vi "Main.vi"(11 "Module Admin":refnum<class "Delacor_lib_QMH_Cloneable Module Admin.lvclass">) -> ()   [LabVIEW 2020, in "TCP Client.lvlib"]
doc: "This template is based off of the Queued Message Handler design pattern and the Queued Message Handler project template that ships with LabVIEW.\n\nThe main difference is that the queue is private to this module and communication between modules is performed via Broadcast and Request events.\n\nRequest events are wrapped in public API methods and are handled in the Event Handling Loop (EHL) of this VI. Any module can register for Broadcast events sent by this module. The EHL generates messages based on user interface actions.\n\nThe Message Handling Loop (MHL) processes messages generated by the EHL, or by other messages. The messages are string values, so new messages can be added easily to the Message Cases case structure in the MHL. Each message cluster can also provide an optional value for Message Data, which is a variant that can be converted to whatever message-specific data is required.\n_____\nBased on Delacor QMH Project Template 6.0.0.89."
uses:
  TCP Client.lvlib
  <vilib>/Delacor/Delacor QMH/Libraries/Cloneable Module Admin_class/Delacor_lib_QMH_Cloneable Module Admin.lvclass
  C:/Program Files (x86)/National Instruments/LabVIEW 2020/vi.lib/Delacor/Delacor QMH/Libraries/Module Admin_class/Delacor_lib_QMH_Module Admin.lvclass
  Module Data--cluster.ctl
  <vilib>/Delacor/Delacor QMH/Libraries/Cloneable Module Admin_class/Delacor_lib_QMH_Cloneable Module Admin.lvclass/Delacor_lib_QMH_Cloneable Module Admin.ctl
  Stop Argument--cluster.ctl
  <vilib>/Delacor/Delacor QMH/Libraries/Message Queue_class/Delacor_lib_QMH_Message Queue.lvclass/Delacor_lib_QMH_Message Queue.ctl
  <vilib>/Delacor/Delacor QMH/Libraries/Module Admin_class/Delacor_lib_QMH_Module Admin.lvclass/Delacor_lib_QMH_Module Admin.ctl
  <vilib>/Utility/miscctls.llb/LVPointTypeDef.ctl
  <vilib>/Delacor/Delacor QMH/Libraries/Cloneable Module Admin_class/Delacor_lib_QMH_Get Module ID.vi
  <vilib>/Delacor/Delacor QMH/Libraries/Message Queue_class/Delacor_lib_QMH_Enqueue Message (Single).vi
  <vilib>/Delacor/Delacor QMH/Libraries/Module Admin_class/Delacor_lib_QMH_Get External Launch.vi
  <vilib>/Utility/error.llb/Error Cluster From Error Code.vi
  <vilib>/ErrorRing/Error Ring.xnode
  <vilib>/Delacor/Delacor QMH/Libraries/Message Queue_class/Delacor_lib_QMH_Message Queue.lvclass
  Test TCP Server API/TCP Server.lvlib
panel:
  out "Module ID":i32=-1
  out "# of Connections":i32
  out "Recieve":T1 {"Gauge" scale=0.0..10.0; "Slide" scale=0.0..10.0}
  out "error out":errorcluster
  out "Status":string
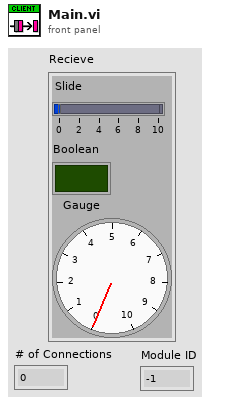
[diagram p1: front panel]
types:
  T1 = cluster{"Slide":dbl, "Boolean":bool, "Gauge":dbl}
  T2 = typedef "TCP Client.lvlib/Request Events--cluster.ctl" = cluster{"Stop Module":refnum<user-event>, "Show Panel":refnum<user-event>, "Hide Panel":refnum<user-event>, "Show Diagram":refnum<user-event>, "Get Module Execution Status":refnum<user-event>, "Connect to TCP Server":refnum<user-event>}
  T3 = typedef "TCP Server.lvlib/Broadcast Events--cluster.ctl" = cluster{"Module Did Init":refnum<user-event>, "Status Updated":refnum<user-event>, "Error Reported":refnum<user-event>, "Module Did Stop":refnum<user-event>, "Update Module Execution Status":refnum<user-event>, "module number":refnum<user-event>}
  T4 = typedef "TCP Client.lvlib/Module Data--cluster.ctl" = cluster{"Status":string}
  T5 = enum32{"invalid lock state", "Not Locked", "Locked (No Password)", "Password-protected"}
  T6 = typedef "TCP Client.lvlib/Stop Argument--cluster.ctl" = cluster{"Module ID":i32, "Origin":string, "Exit via Stop Module Req?":bool, "Wait for Module to stop?":bool}
  T7 = typedef "LVPointTypeDef.ctl" = cluster{"Horizontal":i16, "Vertical":i16}
  T8 = enum32{"Invalid", "Standard", "Closed", "Hidden", "Minimized", "Maximized"}
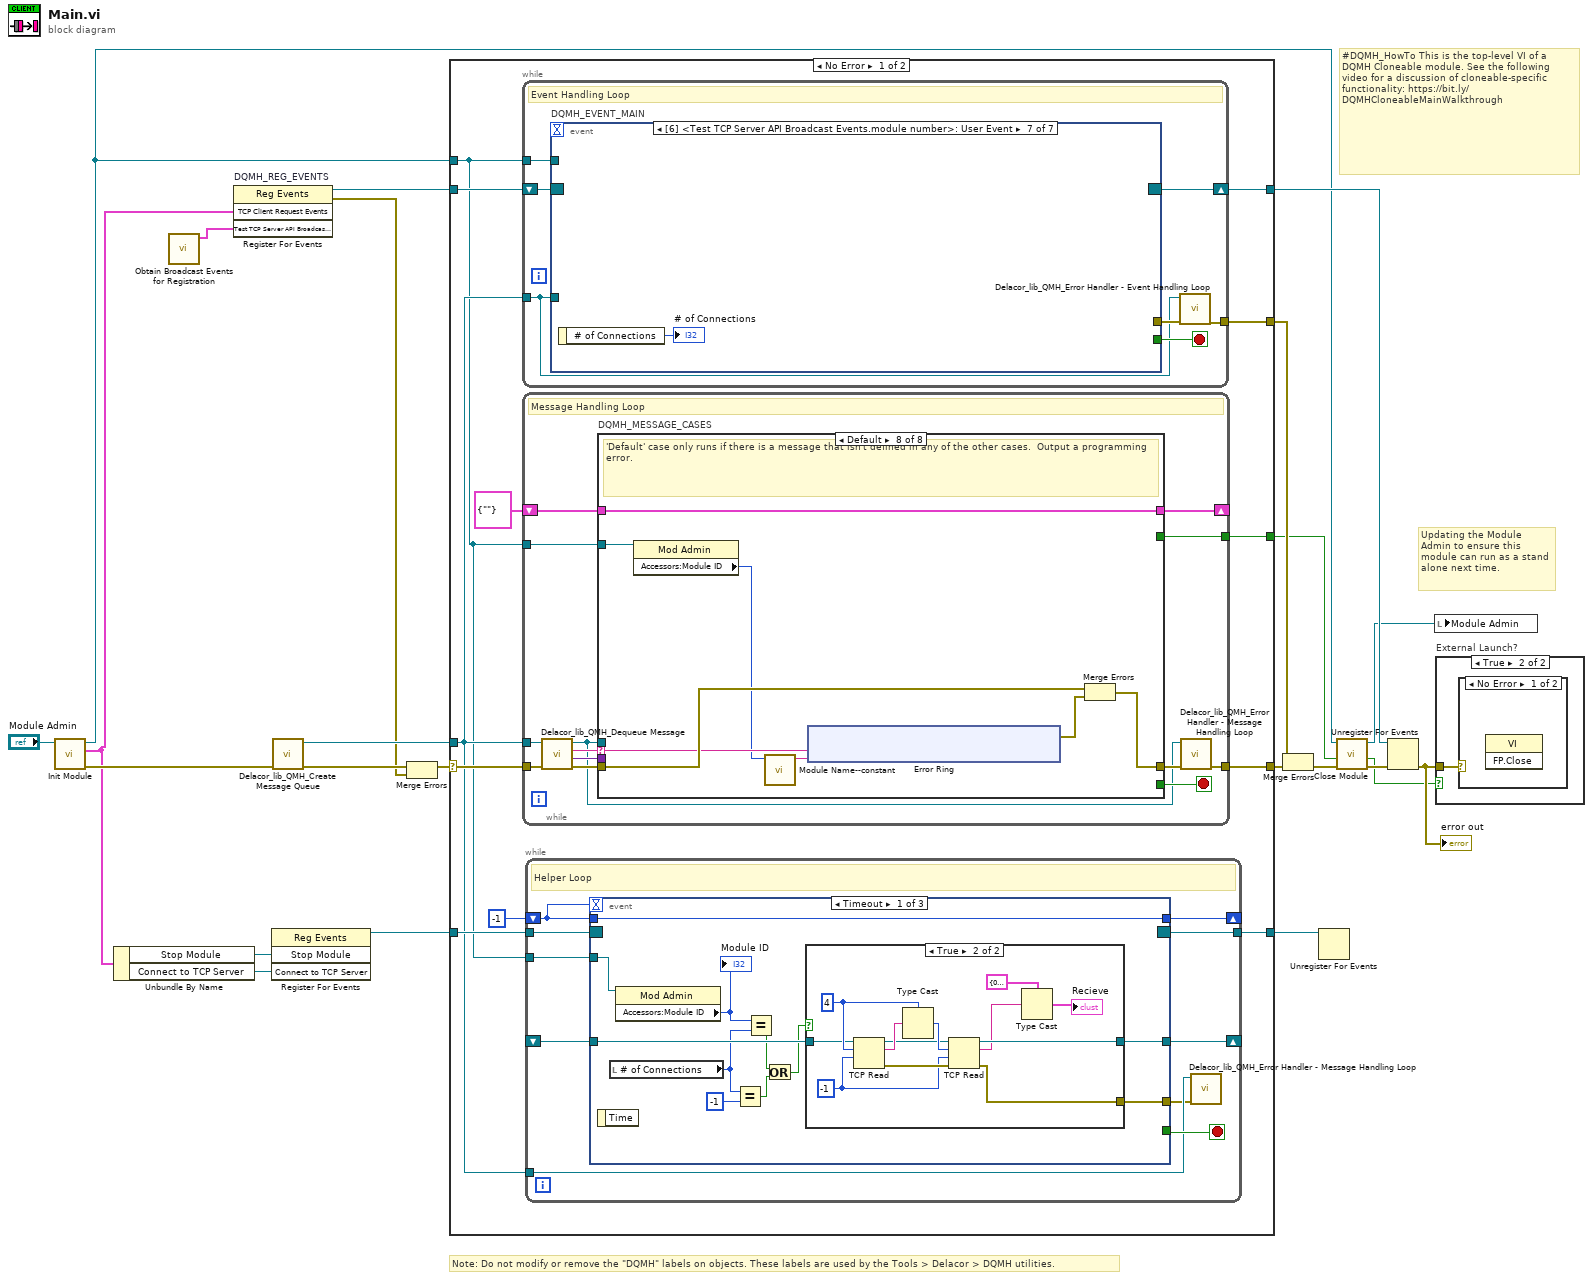
[diagram p0: block diagram]
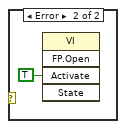
[diagram p3: hidden frame]
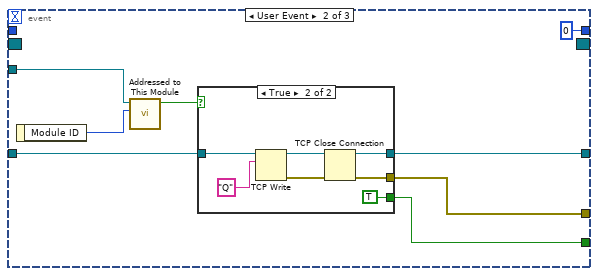
[diagram p5: hidden frame]
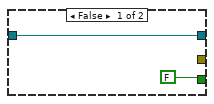
[diagram p6: hidden frame]
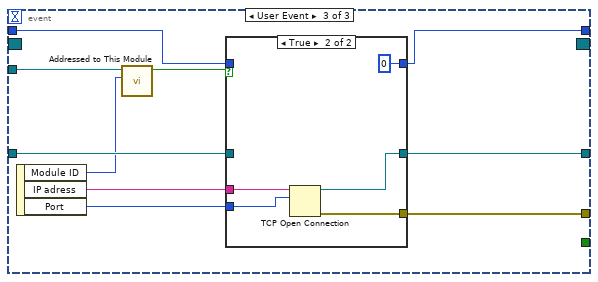
[diagram p7: hidden frame]
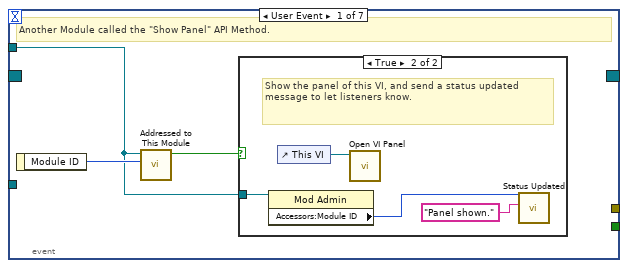
[diagram p9: hidden frame]
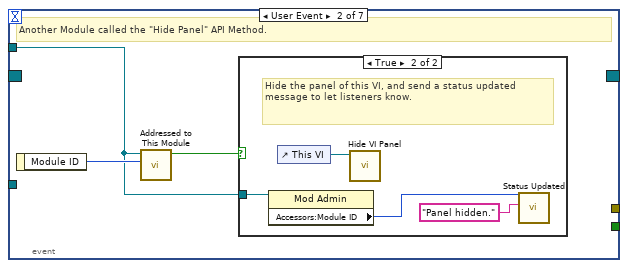
[diagram p11: hidden frame]
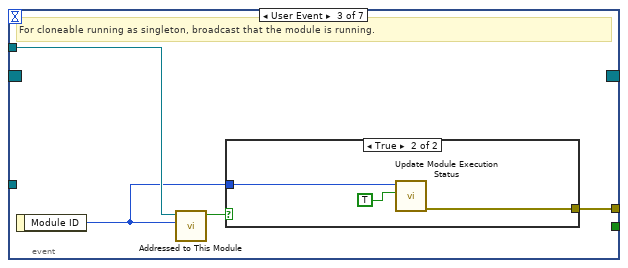
[diagram p13: hidden frame]
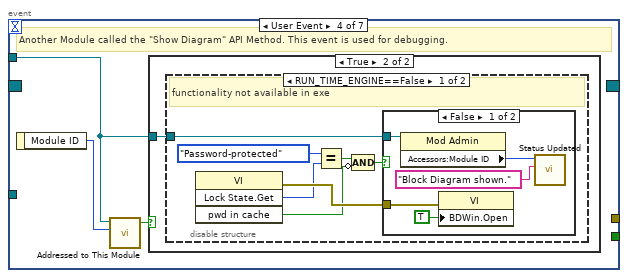
[diagram p15: hidden frame]
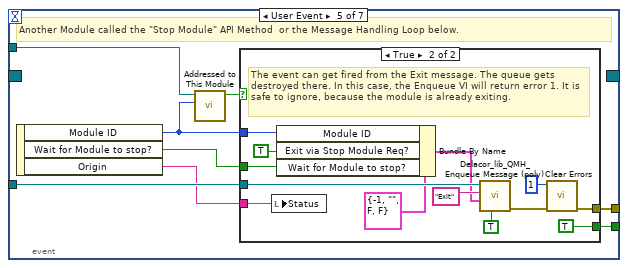
[diagram p19: hidden frame]
diagram:
  # "#DQMH_HowTo This is the top-level VI of a DQMH Cloneable module. See the following video for a discussion of cloneable-specific functionality: https://bit.ly/DQMHCloneableMainWalkthrough"
  # "Note: Do not modify or remove the \"DQMH\" labels on objects. These labels are used by the Tools > Delacor > DQMH utilities."
  # "Updating the Module Admin to ensure this module can run as a stand alone next time."
  n1 = call "Init Module.vi"("Cloneable Module Admin in"="Module Admin") -> ("error out"=w20:errorcluster, "TCP Client Request Events"=w7:T2, "Cloneable Module Admin out"=w11:refnum<class "Delacor_lib_QMH_Cloneable Module Admin.lvclass">)  [unwired: 8 in]
  n2 = Unbundle By Name(w7) -> ("Stop Module"=w6:refnum<user-event>, "Connect to TCP Server"=w3:refnum<user-event>)
  n3 = call "Obtain Broadcast Events for Registration.vi"() -> ("Test TCP Server API Broadcast Events"=w1:T3)  [unwired: 9 in, 2 out]
  n4 = register-events "DQMH_REG_EVENTS"(w7, w1) -> (reference out=w14:refnum<event-registration>, error out=w2:errorcluster)  [unwired: 2 in]
  n5 = register-events(w6, w3) -> (reference out=w5:refnum<event-registration>)  [unwired: 2 in, 1 out]
  n6 = call <vilib>:"Delacor_lib_QMH_Create Message Queue.vi"("error in"=w20) -> ("error out"=w17:errorcluster, "Message Queue"=w13:refnum<class "Delacor_lib_QMH_Message Queue.lvclass">)  [unwired: 9 in]
  n7 = Merge Errors(w17, w2) -> (w16:errorcluster)
  n8 = case shown="No Error" w16 {
    selector: w16 -> [w33 w287]
    tunnel: [w35 w286] -> w21
    tunnel: [w32 w294] -> w15
    tunnel: w14 -> [w30 w294]
    tunnel: w13 -> [w26 w285]
    tunnel: [w34 _] -> w22
    tunnel: w11 -> [w25 w290]
    tunnel: [w29 _] -> w9
    tunnel: w5 -> [w28 w284]
    tunnel: [w27 w284] -> w4
    frame No Error {
      n9 = while {
        tunnel: w26 -> [w104]
        shift-right: [w107] -> w32
        shift-left: w30 -> [w108]
        tunnel: [w109] -> w34
        tunnel: w25 -> [w105]
        stop <- w106 stop-if-true
        # "Event Handling Loop"
        n10 = event "DQMH_EVENT_MAIN" shown="[6] <Test TCP Server API Broadcast Events.module number>: User Event" {
          selector: w108 -> [_ _ _ _ _ _ _]
          dyn-events: [_ _ _ _ _ _ _] -> w107
          timeout: _ -> [_ _ _ _ _ _ _]
          tunnel: [_ _ _ _ w151 _ _] -> w106
          tunnel: w104 -> [_ _ _ _ w154 w170 _]
          tunnel: [_ _ w128 _ w155 w173 _] -> w110
          tunnel: w105 -> [w111 w118 w126 w132 w153 w171 _]
          event User Event {
            # "Another Module called the \"Show Panel\" API Method."
            n11 = event-data() -> ("Module ID"=w112:i32)  [unwired: 1 in]
            n12 = call "Addressed to This Module.vi"("Module ID from Argument"=w112, "Module Admin"=w111) -> ("Addressed to this instance?"=w113:bool)  [unwired: 8 in, 1 out]
            n13 = case shown="True" w113 {
              tunnel: w111 -> [_ w115]
              frame False {
              }
              frame True {
                # "Show the panel of this VI, and send a status updated message to let listeners know."
                n14 = property class="Mod Admin"(reference=w115) -> ("Accessors:Module ID"=w114:i32)  [unwired: 1 in, 2 out]
                n15 = control-ref of="This VI"() -> (w117:refnum<vi>)
                n16 = call "Open VI Panel.vi"("VI"=w117) -> ()  [unwired: 10 in, 1 out]
                n17 = call "Status Updated.vi"("Status"="Panel shown." ("format string"), "Module ID"=w114) -> ()  [unwired: 9 in, 1 out]
              }
            }
          }
          event User Event {
            # "Another Module called the \"Hide Panel\" API Method."
            n18 = event-data() -> ("Module ID"=w119:i32)  [unwired: 1 in]
            n19 = call "Addressed to This Module.vi"("Module ID from Argument"=w119, "Module Admin"=w118) -> ("Addressed to this instance?"=w120:bool)  [unwired: 8 in, 1 out]
            n20 = case shown="True" w120 {
              tunnel: w118 -> [_ w122]
              frame False {
              }
              frame True {
                # "Hide the panel of this VI, and send a status updated message to let listeners know."
                n21 = property class="Mod Admin"(reference=w122) -> ("Accessors:Module ID"=w121:i32)  [unwired: 1 in, 2 out]
                n22 = control-ref of="This VI"() -> (w124:refnum<vi>)
                n23 = call "Hide VI Panel.vi"("VI"=w124) -> ()  [unwired: 10 in, 1 out]
                n24 = call "Status Updated.vi"("Status"="Panel hidden." ("format string"), "Module ID"=w121) -> ()  [unwired: 9 in, 1 out]
              }
            }
          }
          event User Event {
            # "For cloneable running as singleton, broadcast that the module is running."
            n25 = event-data() -> ("Module ID"=w125:i32)  [unwired: 1 in]
            n26 = call "Addressed to This Module.vi"("Module ID from Argument"=w125, "Module Admin"=w126) -> ("Addressed to this instance?"=w127:bool)  [unwired: 8 in, 1 out]
            n27 = case shown="True" w127 {
              tunnel: [_ w131] -> w128
              tunnel: w125 -> [_ w130]
              frame False {
              }
              frame True {
                n28 = call "Update Module Execution Status.vi"("Running?"=TRUE, "Module ID"=w130) -> ("error out"=w131:errorcluster)  [unwired: 9 in]
              }
            }
          }
          event User Event {
            # "Another Module called the \"Show Diagram\" API Method. This event is used for debugging."
            n29 = event-data() -> ("Module ID"=w133:i32)  [unwired: 1 in]
            n30 = call "Addressed to This Module.vi"("Module ID from Argument"=w133, "Module Admin"=w132) -> ("Addressed to this instance?"=w134:bool)  [unwired: 8 in, 1 out]
            n31 = case shown="True" w134 {
              tunnel: w132 -> [_ w135]
              frame False {
              }
              frame True {
                n32 = disable-structure shown="RUN_TIME_ENGINE==False" {
                  disable-tunnel: w135 -> [w136 _]
                  frame condition #0 (active) {
                    # "functionality not available in exe"
                    n33 = invoke class="VI" method="Lock State.Get"() -> (error out=w142:errorcluster, "Get Lock State"=w141:T5, "pwd in cache"=w138:bool)  [unwired: 4 in, 1 out]
                    n34 = Equal?(x=T5."Password-protected", y=w141) -> (x = y?=w139:bool)
                    n35 = Compound Arithmetic op=AND(w139, invert w138) -> (w137:bool)
                    n36 = case shown="False" w137 {
                      tunnel: w142 -> [w147 _]
                      tunnel: w136 -> [w144 _]
                      frame False {
                        n37 = property class="Mod Admin"(reference=w144) -> ("Accessors:Module ID"=w143:i32)  [unwired: 1 in, 2 out]
                        n38 = property class="VI"(error in=w147, "BDWin.Open"=TRUE ("Block Diagram Window:Open")) -> ()  [unwired: 1 in, 2 out]
                        n39 = call "Status Updated.vi"("Status"="Block Diagram shown." ("format string"), "Module ID"=w143) -> ()  [unwired: 9 in, 1 out]
                      }
                      frame True {
                        # "Password-protected VI, and the password is not in the cache. Do not show the diagram."
                      }
                    }
                  }
                  frame condition #1 {
                  }
                }
              }
            }
          }
          event User Event {
            # "Another Module called the \"Stop Module\" API Method  or the Message Handling Loop below."
            n40 = event-data() -> ("Module ID"=w149:i32, "Wait for Module to stop?"=w150:bool, "Origin"=w148:string)  [unwired: 1 in]
            n41 = call "Addressed to This Module.vi"("Module ID from Argument"=w149, "Module Admin"=w153) -> ("Addressed to this instance?"=w152:bool)  [unwired: 8 in, 1 out]
            n42 = case shown="True" w152 {
              tunnel: [_ w167] -> w155
              tunnel: w154 -> [_ w163]
              tunnel: [_ TRUE] -> w151
              tunnel: w150 -> [_ w158]
              tunnel: w149 -> [_ w160]
              tunnel: w148 -> [_ w156]
              frame False {
              }
              frame True {
                # "The event can get fired from the Exit message. The queue gets destroyed there. In this case, the Enqueue VI will return error 1. It is safe to ignore, because the module is already exiting."
                n43 = local write "Status"(w156) -> ()
                n44 = Bundle By Name(cluster=T6 {"Module ID"=-1, "Origin"="", "Exit via Stop Module Req?"=FALSE, "Wait for Module to stop?"=FALSE} ("Stop Argument"), "Module ID"=w160, "Exit via Stop Module Req?"=TRUE, "Wait for Module to stop?"=w158) -> (w157:T6)
                n45 = call-poly <vilib>:"Delacor_lib_QMH_Enqueue Message (poly).vi"("Priority Message? (F)"=TRUE, "Message Data"=w157, "Message"="Exit", "Message Queue in"=w163) -> ("error out"=w168:errorcluster)  [unwired: 6 in, 1 out]
                n46 = call <vilib>:"Clear Errors.vi"("error in (no error)"=w168, "specific error code to clear (0: all)"=1) -> ("error out"=w167:errorcluster)  [unwired: 4 in, 1 out]
              }
            }
          }
          event Panel Close? {
            w172 = TRUE  # Discard the event, the MHL is responsible for closing and stopping this VI.
            # "Hide the panel or send the 'Exit' message if the user clicks the 'X' on the module main VI panel."
            n47 = event-data() -> ()  [unwired: 1 in, 1 out]
            n48 = property class="Mod Admin"(reference=w171) -> ("Accessors:External Launch"=w169:bool)  [unwired: 1 in, 2 out]
            n49 = case shown="True" w169 {
              tunnel: w170 -> [_ w177]
              tunnel: [_ w178] -> w173
              frame True {
                # "If externally launched, clicking the 'X' hides the panel, but doesn't close it."
                n50 = control-ref of="This VI"() -> (w174:refnum<vi>)
                n51 = call "Hide VI Panel.vi"("VI"=w174) -> ()  [unwired: 10 in, 1 out]
              }
              frame False {
                # "If run as a stand-alone VI, clicking the panel 'X' stops the VI."
                n52 = call-poly <vilib>:"Delacor_lib_QMH_Enqueue Message (poly).vi"("Priority Message? (F)"=TRUE, "Message"="Exit", "Message Queue in"=w177) -> ("error out"=w178:errorcluster)  [unwired: 7 in, 1 out]
              }
            }
            n53 = event-data("Discard?"=w172) -> ()  [unwired: 1 in, 1 out]
          }
          event User Event {
            n54 = event-data() -> ("# of Connections"=→"# of Connections":i32)  [unwired: 1 in]
          }
        }
        n55 = call-dynamic "Delacor_lib_QMH_Error Handler - Event Handling Loop.vi"("error in"=w110, "Message Queue in"=w104) -> ("dup error in"=w109:errorcluster)  [unwired: 8 in, 1 out]
      }
      n56 = while {
        tunnel: w26 -> [w183]
        shift-right: [w187] -> _
        shift-left: T4 {"Status"=""} ("Data Cluster") -> [w188]
        tunnel: w33 -> [w191]
        tunnel: [w189] -> w35
        tunnel: w25 -> [w181]
        tunnel: [w180] -> w29
        stop <- w186 stop-if-true
        # "Message Handling Loop"
        n57 = call-dynamic "Delacor_lib_QMH_Dequeue Message.vi"("error in"=w191, "Message Queue in"=w183) -> ("error out"=w190:errorcluster, "Message Data"=w184:variant, "Message"=w185:string, "Message Queue out"=w182:refnum<class "Delacor_lib_QMH_Message Queue.lvclass">)  [unwired: 6 in]
        n58 = case "DQMH_MESSAGE_CASES" shown="Default" w185 {
          selector: w185 -> [_ _ _ _ _ _ _ w271]
          tunnel: w182 -> [_ _ _ _ w222 _ w261 _]
          tunnel: w190 -> [w211 w215 w218 w220 w231 w244 w267 w273]
          tunnel: [w209 w215 w217 w220 w227 w243 w264 w274] -> w192
          tunnel: w188 -> [w202 w214 w216 w219 w226 w241 w260 w272]
          tunnel: [w201 w214 w216 w219 w226 w241 w260 w272] -> w187
          tunnel: [_ _ _ _ _ _ w259 _] -> w186
          tunnel: w184 -> [_ _ _ _ w225 _ w257 _]
          tunnel: w181 -> [w196 _ _ _ w224 w239 w253 w269]
          tunnel: [_ _ _ _ _ _ w255 _] -> w180
          frame "Initialize" {
            w193 = "Initial Message" ("Initial Message")
            # "Initialize - Any operation that needs to be done before the module can receive messages. Synchronize Caller Events.vi will inform Start Module.vi that the module has launched and is ready to receive messages. Module Did Init.vi will broadcast that the module initialized."
            n59 = call "Synchronize Caller Events.vi"("error in (no error)"=w211, "Module Admin"=w196) -> ("error out"=w210:errorcluster, "Module Admin out"=w195:refnum<class "Delacor_lib_QMH_Cloneable Module Admin.lvclass">)  [unwired: 8 in]
            n60 = property class="Mod Admin"(reference=w195) -> ("Accessors:Module ID"=w198:i32, "Accessors:External Launch"=w197:bool)  [unwired: 1 in, 2 out]
            n61 = call "Module Name--constant.vi"("Module ID"=w198) -> ("Module Name"=w206:string)  [unwired: 10 in]
            n62 = property class="VI"("Front Panel.Title"=w206) -> (reference out=w208:refnum<vi>, error out=w213:errorcluster)  [unwired: 2 in]
            n63 = Select(t=T8."Hidden" ("State"), s=w197, f=T8."Standard" ("State")) -> (s? t:f=w203:T8)
            n64 = invoke class="VI" method="FP.Open"(reference=w208, error in=w213, "State"=w203) -> (reference out=w207:refnum<vi>, error out=w212:errorcluster)  [unwired: 2 in, 3 out]
            n65 = call "Module Name--constant.vi"("Module ID"=w198) -> ("Module Name"=w199:string)  [unwired: 10 in]
            n66 = Bundle By Name(cluster=w202, "Status"=w193) -> (w201:T4)
            n67 = invoke class="VI" method="FP.Center"(reference=w207, error in=w212) -> ()  [unwired: 1 in, 3 out]
            n68 = property on="Pane" class="Pane"("Origin"=T7 {"Horizontal"=0, "Vertical"=0}) -> ()  [unwired: 2 in, 2 out]
            n69 = call "Module Did Init.vi"("error in (no error)"=w210, "Initialized?"=TRUE, "Origin"=w199, "Module ID"=w198) -> ("error out"=w209:errorcluster)  [unwired: 7 in]
            "Status" <- w193
          }
          frame "---Module Specific---" {
            # "Separator -- The following cases handle messages specific to this Module."
          }
          frame "---Copy This Frame---" {
            # "Duplicate this frame when creating new messages.  Change this comment in the duplicated frame to describe this message."
            n70 = Merge Errors(w218) -> (w217:errorcluster)
          }
          frame "---Exit and Error Handling---" {
            # "Separator - the following cases handle errors and exit messages."
          }
          frame "Error" {
            # "Error - Check the error message data and respond accordingly. This message is sent by the \"Error Handler\" VIs at the end of each loop in this application."
            n71 = property class="Mod Admin"(reference=w224) -> ("Accessors:External Launch"=w223:bool, "Accessors:Module ID"=w221:i32)  [unwired: 1 in, 2 out]
            n72 = Variant To Data(error in=w231, type=errorcluster {"status"=FALSE, "code"=0, "source"=""} ("error constant"), Variant=w225) -> (data=w232:errorcluster, error out=w229:errorcluster)
            n73 = call "Error Reported.vi"("Error"=w232, "Module ID"=w221) -> ()  [unwired: 9 in, 1 out]
            n74 = case shown="False" w223 {
              tunnel: [w237 _] -> w228
              tunnel: w222 -> [w235 _]
              tunnel: w232 -> [w236 _]
              frame False {
                # "If the module is running standalone, then pop up an error dialog and call the \"Exit\" message."
                n75 = call <vilib>:"Simple Error Handler.vi"("error in (no error)"=w236) -> ()  [unwired: 4 in, 5 out]
                n76 = call-poly <vilib>:"Delacor_lib_QMH_Enqueue Message (poly).vi"("Priority Message? (F)"=TRUE, "Message"="Exit", "Message Queue in"=w235) -> ("error out"=w237:errorcluster)  [unwired: 7 in, 1 out]
              }
              frame True {
                # "If the module was launched externally, calling the Error Reported broadcast VI is the only action performed by the \"Error\" message. The module's caller can then process the error appropriately."
              }
            }
            n77 = Merge Errors(w229, w228) -> (w227:errorcluster)
            n78 = local write "error out"(w227) -> ()
          }
          frame "Simulate MHL Error" {
            # "#DQMH_HowTo The 'Simulate MHL Error' button  illustrates how the MHL handles errors. This event is instructional in nature and can be removed."
            # "Simulate an error occurring at the MHL"
            n79 = property class="Mod Admin"(reference=w239) -> ("Accessors:Module ID"=w240:i32)  [unwired: 1 in, 2 out]
            n80 = call "Module Name--constant.vi"("Module ID"=w240) -> ("Module Name"=w238:string)  [unwired: 10 in]
            n81 = xnode "Error Ring"("parameter 0"=w238) -> ("error out"=w242:errorcluster)
            n82 = Merge Errors(w244, w242) -> (w243:errorcluster)
          }
          frame "Exit" {
            w258 = 91  # 91: not all Exit messages will have an argument
            w259 = TRUE  # Stop the VI
            # "Release the message queue reference"
            # "#CodeNeeded - Add any required cleanup code here."
            # "Exit - Exit the application."
            n83 = Variant To Data(error in=w267, type=T6 {"Module ID"=-1, "Origin"="", "Exit via Stop Module Req?"=FALSE, "Wait for Module to stop?"=FALSE} ("Stop Argument"), Variant=w257) -> (data=w254:T6, error out=w262:errorcluster)
            n84 = call <vilib>:"Clear Errors.vi"("error in (no error)"=w262, "specific error code to clear (0: all)"=w258) -> ("error out"=w266:errorcluster)  [unwired: 4 in, 1 out]
            n85 = control-ref of="This VI"() -> (w252:refnum<vi>)
            n86 = call-dynamic "Delacor_lib_QMH_Release Message Queue.vi"("error in"=w266, "Message Queue"=w261) -> ("error out"=w265:errorcluster)  [unwired: 9 in]
            n87 = call "Handle Exit.vi"("Stop Argument"=w254, "Module Admin in"=w253, "VI reference"=w252) -> ("error out"=w263:errorcluster, "Wait for Stop?"=w255:bool)  [unwired: 7 in]
            n88 = Merge Errors(w265, w263) -> (w264:errorcluster)
          }
          frame Default {
            # "'Default' case only runs if there is a message that isn't defined in any of the other cases.  Output a programming error."
            n89 = property class="Mod Admin"(reference=w269) -> ("Accessors:Module ID"=w268:i32)  [unwired: 1 in, 2 out]
            n90 = call "Module Name--constant.vi"("Module ID"=w268) -> ("Module Name"=w270:string)  [unwired: 10 in]
            n91 = xnode "Error Ring"("parameter 0"=w271, "parameter 1"=w270) -> ("error out"=w275:errorcluster)
            n92 = Merge Errors(w273, w275) -> (w274:errorcluster)
          }
        }
        n93 = call-dynamic "Delacor_lib_QMH_Error Handler - Message Handling Loop.vi"("error in"=w192, "Message Queue in"=w182) -> ("dup error in"=w189:errorcluster)  [unwired: 8 in, 1 out]
      }
      n94 = while {
        tunnel: w28 -> [w45]
        tunnel: [w43] -> w27
        tunnel: w26 -> [w42]
        tunnel: w25 -> [w41]
        shift-right: [w39] -> _
        shift-left: _ -> [w38]
        shift-right: [w36] -> _
        shift-left: -1 -> [w37]
        stop <- w44 stop-if-true
        # "Helper Loop"
        n95 = event shown="[0] Timeout" {
          selector: w45 -> [_ _ _]
          dyn-events: [_ _ _] -> w43
          timeout: w37 -> [_ _ _]
          tunnel: [_ w73 _] -> w44
          tunnel: w41 -> [w52 w71 w87]
          tunnel: [w55 w77 w94] -> w40
          tunnel: [w53 w74 w93] -> w39
          tunnel: w38 -> [w54 w76 w92]
          tunnel: w37 -> [w56 _ w91]
          tunnel: [w56 0 w90] -> w36
          event Timeout {
            n96 = event-data() -> ()  [unwired: 1 in, 1 out]
            n97 = local read "# of Connections"() -> (w48:i32)
            n98 = property class="Mod Admin"(reference=w52) -> ("Accessors:Module ID"=w51:i32)  [unwired: 1 in, 2 out]
            "Module ID" <- w51
            n99 = Equal?(x=w48, y=-1) -> (x = y?=w47:bool)
            n100 = Equal?(x=w51, y=w48) -> (x = y?=w49:bool)
            n101 = Or(x=w49, y=w47) -> (x .or. y?=w50:bool)
            n102 = case shown="True" w50 {
              tunnel: [_ w63] -> w55
              tunnel: w54 -> [w57 w62]
              tunnel: [w57 w61] -> w53
              frame False {
              }
              frame True {
                w64 = -1
                w65 = 4
                n103 = TCP Read(connection ID=w62, bytes to read=w65, 9:w64) -> (connection ID out=w66:refnum<k5>, data out=w69:string, error out=w68:errorcluster)  [unwired: 1 in, 1 out]
                n104 = Type Cast(type=w65, x=w69) -> (*(type *) &x=w67:i32)
                n105 = TCP Read(connection ID=w66, bytes to read=w67, error in (no error)=w68, 9:w64) -> (connection ID out=w61:refnum<k5>, data out=w58:string, error out=w63:errorcluster)  [unwired: 1 out]
                n106 = Type Cast(type=T1 {"Slide"=0.0, "Boolean"=FALSE, "Gauge"=0.0} ("Recieve"), x=w58) -> (*(type *) &x=→"Recieve":T1)
              }
            }
          }
          event User Event {
            n107 = event-data() -> ("Module ID"=w72:i32)  [unwired: 1 in]
            n108 = call "Addressed to This Module.vi"("Module ID from Argument"=w72, "Module Admin"=w71) -> ("Addressed to this instance?"=w70:bool)  [unwired: 8 in, 1 out]
            n109 = case shown="True" w70 {
              tunnel: [_ w86] -> w77
              tunnel: w76 -> [w79 w82]
              tunnel: [w79 w85] -> w74
              tunnel: [FALSE TRUE] -> w73
              frame False {
              }
              frame True {
                n110 = TCP Write(connection ID=w82, data in="Q") -> (connection ID out=w81:refnum<k5>, error out=w80:errorcluster)  [unwired: 1 in, 2 out]
                n111 = TCP Close Connection(connection ID=w81, error in (no error)=w80) -> (connection ID out=w85:refnum<k5>, error out=w86:errorcluster)  [unwired: 1 out]
              }
            }
          }
          event User Event {
            n112 = event-data() -> ("Module ID"=w88:i32, "IP adress"=w96:string, "Port"=w95:u16)  [unwired: 1 in]
            n113 = call "Addressed to This Module.vi"("Module ID from Argument"=w88, "Module Admin"=w87) -> ("Addressed to this instance?"=w89:bool)  [unwired: 8 in, 1 out]
            n114 = case shown="True" w89 {
              tunnel: w96 -> [_ w103]
              tunnel: w95 -> [_ w102]
              tunnel: [_ w101] -> w94
              tunnel: [w98 w100] -> w93
              tunnel: w92 -> [w98 _]
              tunnel: w91 -> [w97 _]
              tunnel: [w97 0] -> w90
              frame False {
              }
              frame True {
                n115 = TCP Open Connection(address=w103, remote port or service name=w102) -> (connection ID=w100:refnum<k5>, error out=w101:errorcluster)  [unwired: 1 in, 2 out]
              }
            }
          }
        }
        n116 = call-dynamic "Delacor_lib_QMH_Error Handler - Message Handling Loop.vi"("error in"=w40, "Message Queue in"=w42) -> ()  [unwired: 8 in, 2 out]
      }
    }
    frame Error {
      n117 = call "Synchronize Caller Events.vi"("Module Admin"=w290) -> ("Module Admin out"=w289:refnum<class "Delacor_lib_QMH_Cloneable Module Admin.lvclass">)  [unwired: 9 in, 1 out]
      n118 = property class="Mod Admin"(reference=w289) -> ("Accessors:Module ID"=w288:i32)  [unwired: 1 in, 2 out]
      n119 = call-dynamic "Delacor_lib_QMH_Release Message Queue.vi"("error in"=w287, "Message Queue"=w285) -> ("error out"=w286:errorcluster)  [unwired: 9 in]
      n120 = call "Module Name--constant.vi"("Module ID"=w288) -> ("Module Name"=w293:string)  [unwired: 10 in]
      n121 = Format Into String(format string="An error occurred during initialization. %s is no longer running.", w293) -> (resulting string=w291:string)  [unwired: 2 in, 1 out]
      n122 = call "Error Reported.vi"("Additional Information"=w291, "Error"=w286, "Module ID"=w288) -> ()  [unwired: 8 in, 1 out]
    }
  }
  n123 = Merge Errors(w22, w21) -> (w23:errorcluster)
  n124 = Unregister For Events(event registration refnum=w4) -> ()  [unwired: 1 in, 1 out]
  n125 = call "Close Module.vi"("error in"=w23, "Wait for stop?"=w9, "Module Admin in"=w11) -> ("error out"=w19:errorcluster, "External Launch"=w8:bool, "Module Admin out"=w10:refnum<class "Delacor_lib_QMH_Cloneable Module Admin.lvclass">)  [unwired: 6 in]
  n126 = Unregister For Events(event registration refnum=w15, error in=w19) -> (error out=w18:errorcluster)
  "error out" <- w18
  n127 = local write "Module Admin"(w10) -> ()
  n128 = case "External Launch?" shown="True" w8 {
    tunnel: w18 -> [_ w295]
    frame False {
    }
    frame True {
      n129 = case shown="No Error" w295 {
        frame No Error {
          n130 = invoke class="VI" method="FP.Close"() -> ()  [unwired: 3 in, 3 out]
        }
        frame Error {
          n131 = invoke class="VI" method="FP.Open"("Activate"=TRUE ("Activate?")) -> ()  [unwired: 4 in, 5 out]
        }
      }
    }
  }
